vi "Z900_navX_Open_SPI.vi"(8 "error in (no error)":errorcluster, 9 "Clock Rate (Hz)":dbl=2000000.0 format="%_6f", 10 "SPI Bus":T3=enum."SPI MXP", 11 "Update Rate (4Hz-60Hz)":u8=50 min=4 max=60) -> (0 "error out":errorcluster, 3 "navX Device":T1={"Interface"={"Protocol"=enum."SERIAL", "Update Rate (4Hz-60Hz)"=4, "navX Open TypeDef"=variant}, "Notify Packet"=refnum, "Loop VI Refnum"=refnum, "Ready to Close Occurrence Refnum"=refnum} {"Interface"."Update Rate (4Hz-60Hz)" min=4 max=60 step=1})   [LabVIEW 2016, in "navX Library v2.lvlib"]
doc: "This VI opens the navX over SPI. You must open a reference before using any other VIs on this palette. After you open a reference to the navX, you can use the other navX VIs to access and monitor the navX device."
uses:
  navX Library v2.lvlib
  <vilib>/Rock Robotics/SystemInterfaces/spilib/spi_bus.ctl
  TypeDefs/Z900_navX_DeviceTypeDef.ctl
  TypeDefs/Z900_navX_ProtocolTypeDef.ctl
  TypeDefs/Z900_navX_NotifyPacketTypeDef.ctl
  TypeDefs/Z900_navX_ActionTypeDef.ctl
  TypeDefs/navX Open TypeDefs/Z900_navX_OpenTypeDef_SPI.ctl
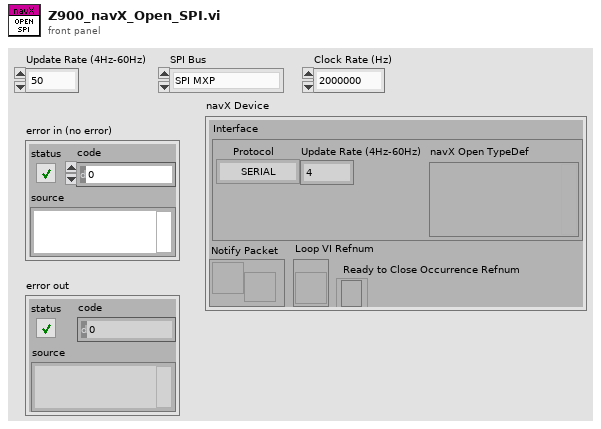
[diagram p1: front panel]
types:
  T1 = typedef "navX Library v2.lvlib/Z900_navX_DeviceTypeDef.ctl" = cluster{"Interface":cluster{"Protocol":T2, "Update Rate (4Hz-60Hz)":u8, "navX Open TypeDef":variant}, "Notify Packet":refnum<notifier>, "Loop VI Refnum":refnum<vi>, "Ready to Close Occurrence Refnum":refnum<k4>}
  T2 = typedef "navX Library v2.lvlib/Z900_navX_ProtocolTypeDef.ctl" = enum16{"SERIAL", "I2C", "SPI"}
  T3 = typedef "spi_bus.ctl" = enum16{"SPI On-Board, CS0", "SPI On-Board, CS1", "SPI On-Board, CS2", "SPI On-Board, CS3", "SPI MXP", "Invalid"}
  T4 = typedef "navX Library v2.lvlib/Z900_navX_OpenTypeDef_SPI.ctl" = cluster{"SPI Bus":T3, "Clock Rate (Hz)":dbl}
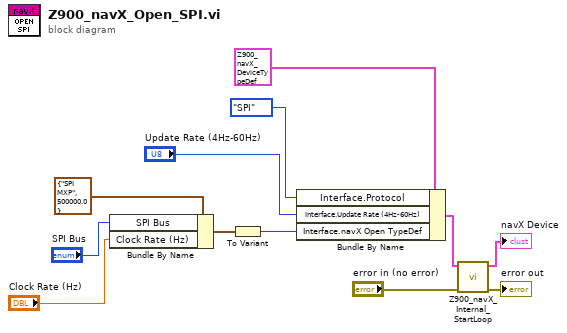
[diagram p0: block diagram]
diagram:
  n1 = Bundle By Name(cluster=T4 {"SPI Bus"=enum."SPI MXP", "Clock Rate (Hz)"=500000.0} ("navX SPI Open"), "SPI Bus"="SPI Bus", "Clock Rate (Hz)"="Clock Rate (Hz)") -> (w9:T4)
  n2 = To Variant(anything=w9) -> (Variant=w8:variant)
  n3 = Bundle By Name(cluster=T1 {"Interface"={"Protocol"=enum."SERIAL", "Update Rate (4Hz-60Hz)"=0, "navX Open TypeDef"=variant}, "Notify Packet"=refnum, "Loop VI Refnum"=refnum, "Ready to Close Occurrence Refnum"=refnum} ("navX Device"), "Interface.Protocol"=Z900_navX_ProtocolTypeDef."SPI", "Interface.Update Rate (4Hz-60Hz)"="Update Rate (4Hz-60Hz)", "Interface.navX Open TypeDef"=w8) -> (w5:T1)
  n4 = call "Z900_navX_Internal_StartLoop.vi"("error in (no error)"="error in (no error)", "navX Device"=w5) -> ("error out"=→"error out":errorcluster, "navX Device"=→"navX Device":T1)  [unwired: 8 in]
